vi "P9P14T_Merge_Cluster.vi"(1 "P9/P14-Magnet-Control":T1 {"Approach" items=["Linear", "NoOvershoot", "Oscillate"]}, 2 "P9/P14-Magnet Status":T2 {"Magnet Status" items=["MagnetUnknown"=0, "StablePersistent"=1, "WarmingSwitch"=2, "CoolingSwitch"=3, "StableDriven"=4, "Iterating"=5, "Charging"=6, "Discharging"=7, "CurrentError"=8, "MagnetFailure"=15]}) -> (0 "P9/P14-Magnet-Cluster":T3 {"Magnet Status" items=["MagnetUnknown"=0, "StablePersistent"=1, "WarmingSwitch"=2, "CoolingSwitch"=3, "StableDriven"=4, "Iterating"=5, "Charging"=6, "Discharging"=7, "CurrentError"=8, "MagnetFailure"=15]; "Approach" items=["Linear", "NoOvershoot", "Oscillate"]})   [LabVIEW 2019]
uses:
  PPMS/P9_P14_Magnet-cluster.ctl
  PPMS/P9P14_Magnet_Status.ctl
  PPMS/P9P14_Magnet_Control.ctl
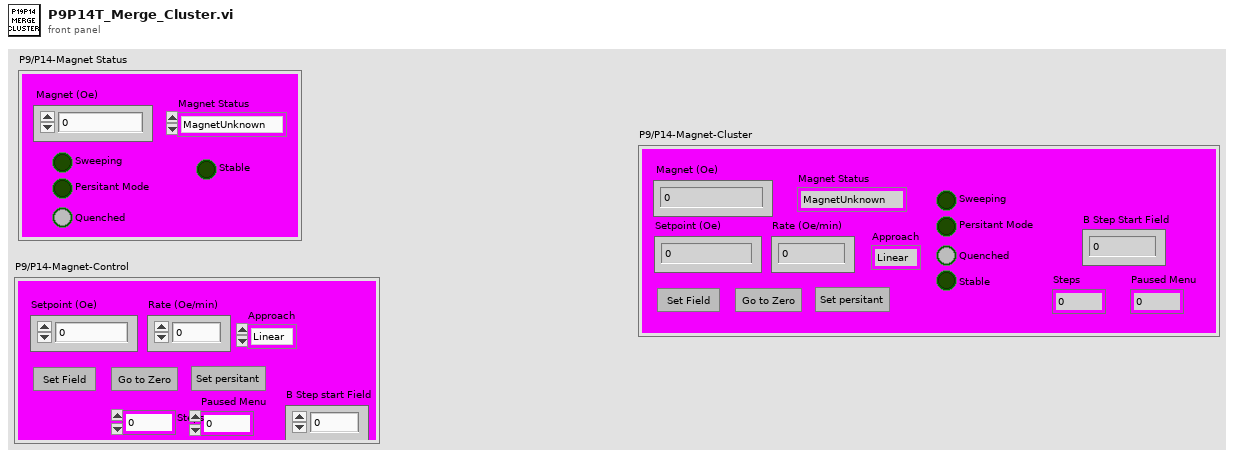
[diagram p1: front panel]
types:
  T1 = typedef "P9P14_Magnet_Control.ctl" = cluster{"Setpoint (Oe)":dbl, "Rate (Oe/min)":dbl, "Set Field":bool, "Go to zero":bool, "Set Persitant/non-pers":bool, "Approach":i32, "Steps":dbl, "Paused Menu":dbl, "B Step start Field":dbl}
  T2 = typedef "P9P14_Magnet_Status.ctl" = cluster{"Magnet (Oe)":dbl, "Magnet Status":i32, "Sweeping":bool, "Quenched":bool, "Persitant Mode ":bool, "Stable":bool}
  T3 = typedef "P9_P14_Magnet-cluster.ctl" = cluster{"Magnet (Oe)":dbl, "Setpoint (Oe)":dbl, "Rate (Oe/min)":dbl, "Set Field":bool, "Go to zero":bool, "Set Persitant/non-pers":bool, "Approach":i32, "Magnet Status":i32, "Sweeping":bool, "Quenched":bool, "Persitant Mode ":bool, "Stable":bool, "Steps":dbl, "Paused Menu":dbl, "B Step Start Field":dbl}
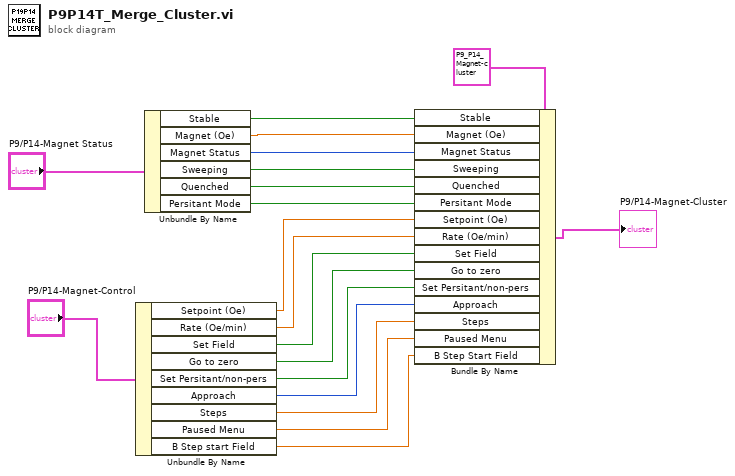
[diagram p0: block diagram]
diagram:
  n1 = Unbundle By Name("P9/P14-Magnet-Control") -> ("Setpoint (Oe)"=w11:dbl, "Rate (Oe/min)"=w10:dbl, "Set Field"=w9:bool, "Go to zero"=w8:bool, "Set Persitant/non-pers"=w7:bool, "Approach"=w6:i32, "Steps"=w4:dbl, "Paused Menu"=w3:dbl, "B Step start Field"=w2:dbl)
  n2 = Unbundle By Name("P9/P14-Magnet Status") -> ("Stable"=w1:bool, "Magnet (Oe)"=w17:dbl, "Magnet Status"=w16:i32, "Sweeping"=w15:bool, "Quenched"=w14:bool, "Persitant Mode"=w13:bool)
  n3 = Bundle By Name(cluster=T3 {"Magnet (Oe)"=0.0, "Setpoint (Oe)"=0.0, "Rate (Oe/min)"=0.0, "Set Field"=FALSE, "Go to zero"=FALSE, "Set Persitant/non-pers"=FALSE, "Approach"=0, "Magnet Status"=0, "Sweeping"=FALSE, "Quenched"=FALSE, "Persitant Mode "=FALSE, "Stable"=FALSE, "Steps"=0.0, "Paused Menu"=0.0, "B Step Start Field"=0.0} ("P9/P14-Magnet-Cluster 2"), "Stable"=w1, "Magnet (Oe)"=w17, "Magnet Status"=w16, "Sweeping"=w15, "Quenched"=w14, "Persitant Mode"=w13, "Setpoint (Oe)"=w11, "Rate (Oe/min)"=w10, "Set Field"=w9, "Go to zero"=w8, "Set Persitant/non-pers"=w7, "Approach"=w6, "Steps"=w4, "Paused Menu"=w3, "B Step Start Field"=w2) -> (→"P9/P14-Magnet-Cluster":T3)
